vi "Find Refs.vi"(7 "Actor in":refnum<class "Actor.lvclass">) -> (0 "Error out":errorcluster, 2 "Refs":T1)   [LabVIEW 2025, in "_Template.lvlib" / "Templates.lvlib" / "TEMPLATE Actor.lvlib" / "TEMPLATE Actor.lvlib" / "TEMPLATE Refs.lvlib"]
uses:
  TEMPLATE Refs.lvlib
  jettl/jettl/Actor/Actor.lvclass
  Refs.ctl
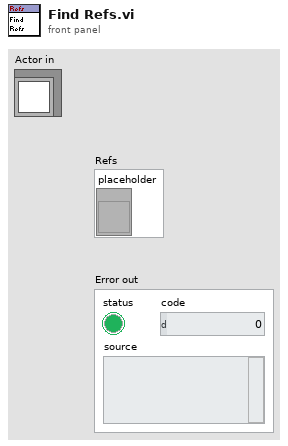
[diagram p1: front panel]
types:
  T1 = typedef "_Template.lvlib/Templates.lvlib/TEMPLATE Actor.lvlib/TEMPLATE Actor.lvlib/TEMPLATE Refs.lvlib/Refs.ctl" = cluster{"placeholder":refnum<vi>}
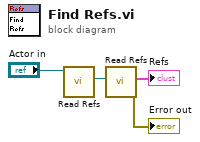
[diagram p0: block diagram]
diagram:
  n1 = call-dynamic "Read Refs.vi"("Actor in"="Actor in") -> ("Refs"=w4:refnum<class "Refs.lvclass">)  [unwired: 10 in]
  n2 = call "Read Refs.vi"("Refs"=w4) -> ("Error out"=→"Error out":errorcluster, "Refs"=→"Refs":T1)  [unwired: 9 in]
